vi "Update-status.vi"(6 "Status":T1, 8 "error in (no error)":errorcluster, 11 "Object ref in":T2) -> (0 "error out":errorcluster, 3 "Object ref out":T2)   [LabVIEW 2013, in "SLMControl.lvlib" / "SC-Main.lvclass"]
uses:
  SC-Main.lvclass
  Object-reference.ctl
  Application-status.ctl
  UI/Control-names.ctl
  SC-Main.lvclass/SC-Main.ctl
  Read UI.vi
  Read Client.vi
  Write Status.vi
  UI/Set-control-string.vi
  UI/SC-UI.lvclass
  Client/Sources/SC-Client.lvclass
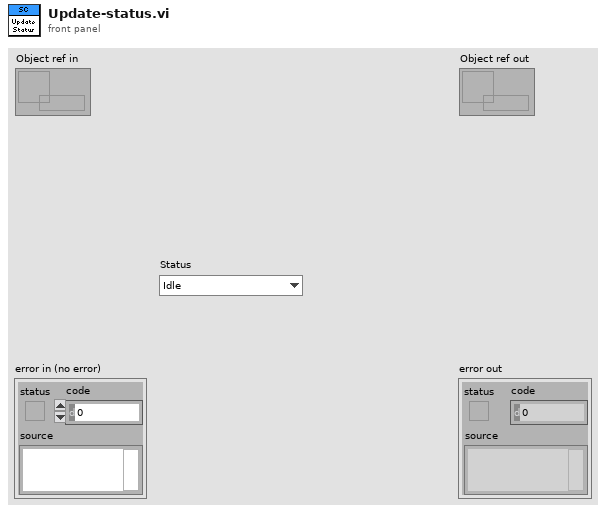
[diagram p1: front panel]
types:
  T1 = typedef "SLMControl.lvlib/SC-Main.lvclass/Application-status.ctl" = enum16{"Idle", "Initialized", "Configured", "Activated", "Started", "Paused", "Stopped", "Reset", "Error", "Exited"}
  T2 = typedef "SLMControl.lvlib/SC-Main.lvclass/Object-reference.ctl" = refnum<data-value>
  T3 = typedef "SLMControl.lvlib/SC-UI.lvclass/Control-names.ctl" = enum16{"Com-in", "Com-out", "Help", "Status", "Load configuration", "Save configuration", "Load lasing files", "Load deposition files", "Clear", "Files", "Activate", "Execute", "Abort", "Options", "Current layer", "Current iteration", "Last elapsed time", "Deposition status", "Lasing job", "Status LEDs", "Exiting led", "Initialized led", "Files loaded led", "Activated led", "Executing led", "Deposition led", "Lasing job led", "Lasing led"}
  T4 = typedef "SLMControl.lvlib/SC-UI.lvclass/Panes-reference.ctl" = refnum<data-value>
  T5 = typedef "SLMControl.lvlib/SC-Client.lvclass/Object-reference.ctl" = refnum<data-value>
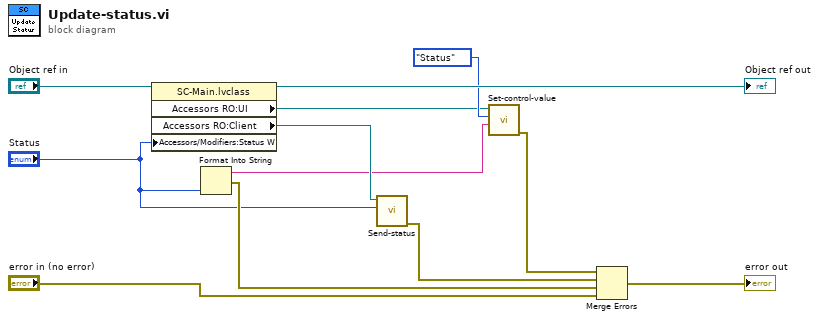
[diagram p0: block diagram]
diagram:
  n1 = property class="SC-Main.lvclass"(reference="Object ref in", "Accessors/Modifiers:Status W"="Status") -> (reference out=→"Object ref out":T2, "Accessors RO:UI"=w5:T4, "Accessors RO:Client"=w9:T5)  [unwired: 1 in, 1 out]
  n2 = Format Into String("Status") -> (resulting string=w3:string, error out=w4:errorcluster)  [unwired: 3 in]
  n3 = call "Send-status.vi"("Status"="Status", "Client in"=w9) -> ("error out"=w8:errorcluster)  [unwired: 8 in, 1 out]
  n4 = call-poly "Set-control-value.vi"("Value"=w3, "Control name"=Control-names."Status", "Panes in"=w5) -> ("error out"=w6:errorcluster)  [unwired: 7 in, 1 out]
  n5 = Merge Errors(w6, w8, w4, "error in (no error)") -> (→"error out":errorcluster)
